vi "PlotSingleCube.vi"() -> ()   [LabVIEW 2014]
uses:
  TypeDefs/PowerSpeed.ctl
  TypeDefs/RectHatch.ctl
panel:
  in  "RectHatch":T1={"Width"=10.0, "Height"=10.0, "Angle"=45.0, "OffX"=0.1, "OffY"=0.1, "Spacing"=0.1, "IslandSize"=0.1} {"IslandSize" format="%#_13g"; "Spacing" format="%#_13g"; "OffY" format="%#_13g"; "OffX" format="%#_13g"; "Height" format="%#_13g"; "Width" format="%#_13g"}
  in  "EndLayer":u32=170
  in  "Display":T2={"Mode"=enum."Inherit Value", "PointSize"=1.0, "LineWidth"=1.0}
  in  "HighPower":dbl=500.0
  in  "StartLayer":u32=170
  in  "HatchPow":T3={"Power"=300.0, "Mark Speed"=400.0, "Jump Speed"=1000.0, "JumpPower"=0.0}
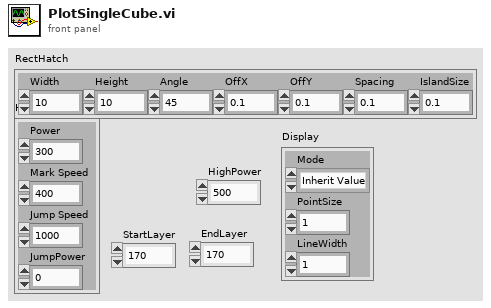
[diagram p1: front panel]
types:
  T1 = typedef "RectHatch.ctl" = cluster{"Width":dbl, "Height":dbl, "Angle":sgl, "OffX":dbl, "OffY":dbl, "Spacing":dbl, "IslandSize":dbl}
  T2 = cluster{"Mode":enum16{"Inherit Value", "Points", "Wireframe", "Polygons"}, "PointSize":sgl, "LineWidth":sgl}
  T3 = typedef "PowerSpeed.ctl" = cluster{"Power":dbl, "Mark Speed":dbl, "Jump Speed":dbl, "JumpPower":dbl}
  T4 = typedef "PathSupreme.ctl" = cluster{"VelocityProfiles":T5[], "Path":T6}
  T5 = typedef "VelocityProfile.ctl" = cluster{"ID":u32, "Velocity":dbl, "Mode":string, "tV1":u32, "tV2":u32, "tL1":u32, "tL2":u32}
  T6 = typedef "PathCut.ctl" = cluster{"Type":string, "Tag":string, "Segments":T7[]}
  T7 = typedef "Segment.ctl" = cluster{"SegmentID":u16, "Power":sgl, "idxVelocityProfile":u16, "End":cluster{"X":sgl, "Y":sgl}}
  T8 = typedef "Point3D.ctl" = cluster{"X":sgl, "Y":sgl, "Z":sgl}
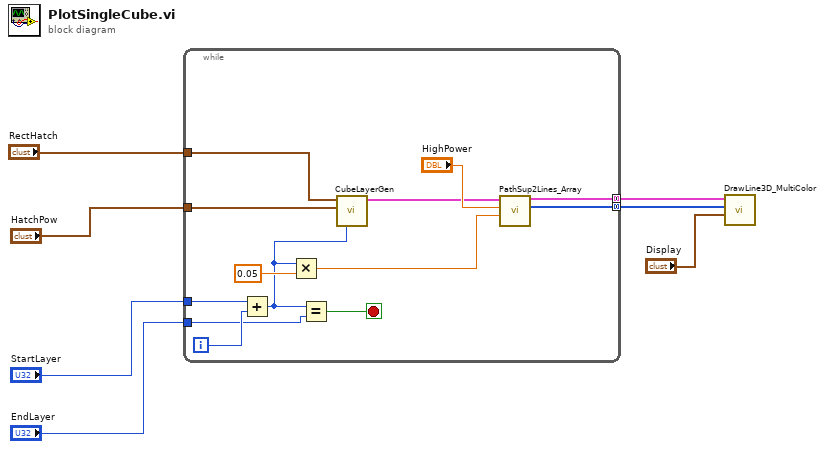
[diagram p0: block diagram]
diagram:
  n1 = while {
    tunnel: [w20] -> w7 mode=concatenating
    tunnel: [w19] -> w6 mode=concatenating
    tunnel: "HatchPow" -> [w10]
    tunnel: "StartLayer" -> [w15]
    tunnel: "EndLayer" -> [w13]
    tunnel: "RectHatch" -> [w8]
    i -> [w14]
    stop <- w16 stop-if-true
    n2 = Add(x=w15, y=w14) -> (x+y=w9:u32)
    n3 = Multiply(x=w9, y=0.05) -> (x*y=w12:dbl)
    n4 = Equal?(x=w9, y=w13) -> (x = y?=w16:bool)
    n5 = call "CubeLayerGen.vi"("Layer"=w9, "HatchPow"=w10, "RectHatch"=w8) -> ("PathSups"=w11:T4[])  [unwired: 8 in]
    n6 = call "PathSup2Lines_Array.vi"("Z"=w12, "HighPower"="HighPower", "PathSupIn"=w11) -> ("Colors"=w19:u32[], "Lines"=w20:cluster{"P0":T8, "P1":T8}[])  [unwired: 7 in]
  }
  n7 = call "DrawLine3D_MultiColor.vi"("Display"="Display", "Colors"=w6, "Lines"=w7) -> ()  [unwired: 9 in]
